vi "Read Latest 2 Values.vi"(8 "error in (no error)":errorcluster, 11 "Ring buffer DVR in":refnum<data-value>) -> (0 "error out":errorcluster, 1 "Values (latest)":u8[](array[numeric]), 2 "Timestamp (latest)":u64, 3 "Ring buffer DVR out":refnum<data-value>, 4 "Timestamp (previous)":u64, 5 "empty buffer? (previous)":bool, 6 "Values (previous)":u8[](array[numeric]), 7 "empty buffer? (latest)":bool)   [LabVIEW 2021, in "Ring Buffer Time Series Data.lvlib"]
uses:
  Ring Buffer Time Series Data.lvlib
  SubVIs/DVR data.ctl
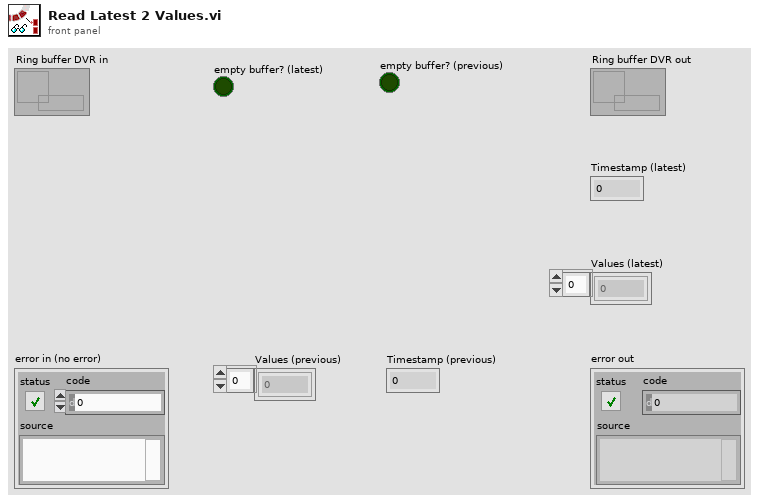
[diagram p1: front panel]
types:
  T1 = typedef "Ring Buffer Time Series Data.lvlib/DVR data.ctl" = cluster{"Timestamps":u64[], "Values":u8[], "#bytes per timestamp":i32, "Index":i32, "Size (#timestamps)":i32, "Full?":bool}
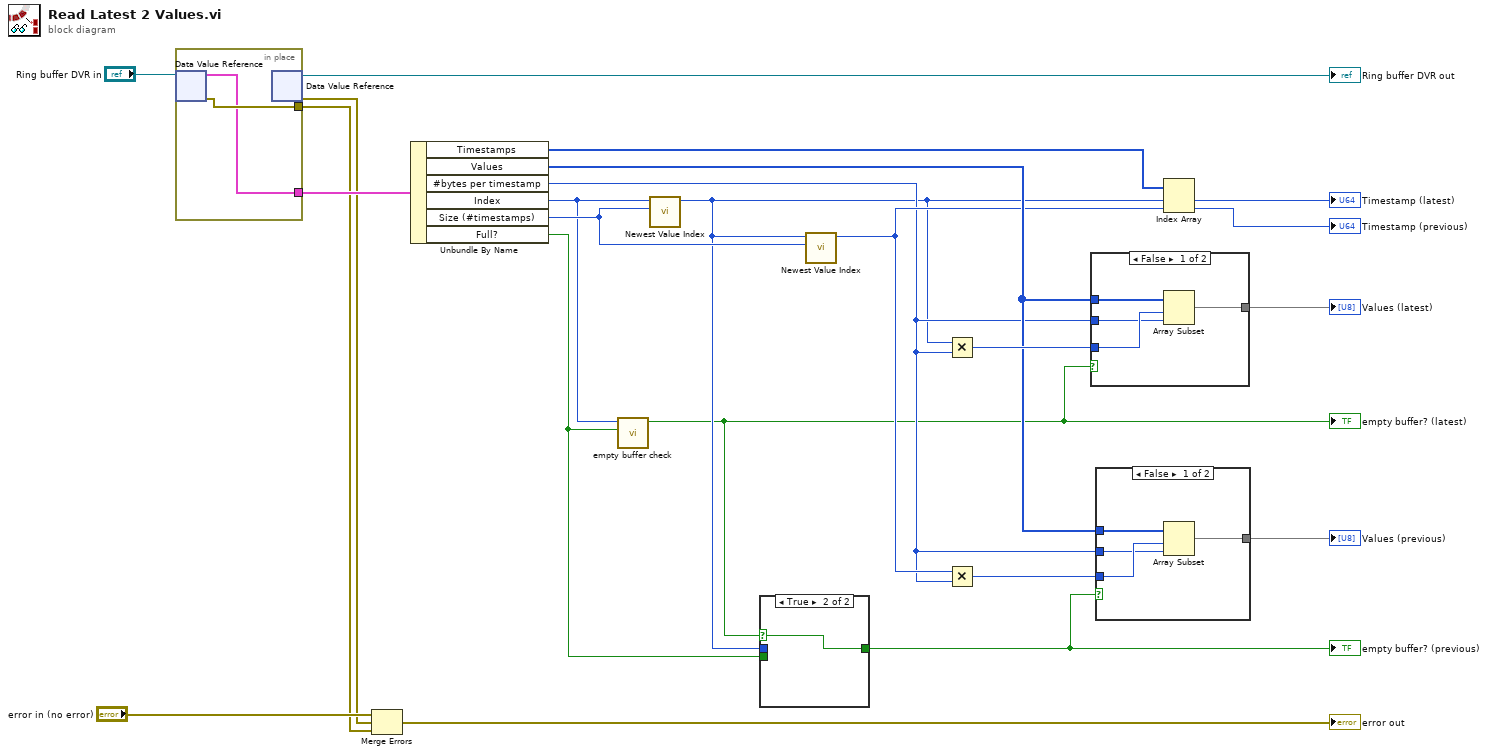
[diagram p0: block diagram]
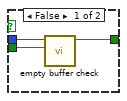
[diagram p2: hidden frame]
diagram:
  n1 = in-place {
    in-place-border: [w25] -> w13
    in-place-border: [w24] -> w17
    n2 = in-place-dvr #1("Ring buffer DVR in") -> (w24:T1, w25:errorcluster)
    n3 = in-place-dvr #1() -> (→"Ring buffer DVR out":refnum<data-value>, w14:errorcluster)  [unwired: 1 in]
  }
  n4 = Merge Errors("error in (no error)", w14, w13) -> (→"error out":errorcluster)
  n5 = Unbundle By Name(w17) -> ("Timestamps"=w16:u64[], "Values"=w10:u8[], "#bytes per timestamp"=w7:i32, "Index"=w5:i32, "Size (#timestamps)"=w12:i32, "Full?"=w4:bool)
  n6 = call "empty buffer check.vi"("Full?"=w4, "Index"=w5) -> ("empty buffer?"=w1:bool)  [unwired: 9 in]
  "empty buffer? (latest)" <- w1
  n7 = call "Newest Value Index.vi"("Size"=w12, "Index"=w5) -> ("Newest value index"=w3:i32)  [unwired: 9 in]
  n8 = case shown="True" w1 {
    selector: w1 -> [_ w29]
    tunnel: w4 -> [w28 _]
    tunnel: w3 -> [w27 _]
    tunnel: [w26 w29] -> w2
    frame False {
      n9 = call "empty buffer check.vi"("Full?"=w28, "Index"=w27) -> ("empty buffer?"=w26:bool)  [unwired: 9 in]
    }
    frame True {
    }
  }
  "empty buffer? (previous)" <- w2
  n10 = call "Newest Value Index.vi"("Size"=w12, "Index"=w3) -> ("Newest value index"=w9:i32)  [unwired: 9 in]
  n11 = Multiply(x=w3, y=w7) -> (x*y=w15:i32)
  n12 = Multiply(x=w9, y=w7) -> (x*y=w8:i32)
  n13 = case shown="False" w1 {
    tunnel: [w33 _] -> w21
    tunnel: w15 -> [w32 _]
    tunnel: w10 -> [w31 _]
    tunnel: w7 -> [w30 _]
    frame False {
      n14 = Array Subset(array=w31, index=w32, length=w30) -> (w33:u8[])
    }
    frame True {
    }
  }
  "Values (latest)" <- w21
  n15 = case shown="False" w2 {
    tunnel: w10 -> [w37 _]
    tunnel: w8 -> [w36 _]
    tunnel: w7 -> [w35 _]
    tunnel: [w34 _] -> w6
    frame False {
      n16 = Array Subset(array=w37, index=w36, length=w35) -> (w34:u8[])
    }
    frame True {
    }
  }
  "Values (previous)" <- w6
  n17 = Index Array(array=w16, index #1=w3, index #2=w9) -> (element #1=→"Timestamp (latest)":u64, element #2=→"Timestamp (previous)":u64)
